vi "Freeze.vi"(8 "Error In":errorcluster, 9 "Waveforms in":waveform(dbl)[](array[waveform]), 10 "Freeze":bool) -> (0 "Error Out":errorcluster, 1 "Waveforms out":waveform(dbl)[](array[waveform]))   [LabVIEW 2017]
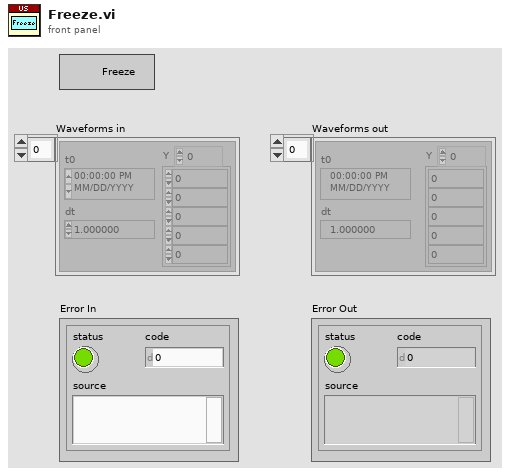
[diagram p1: front panel]
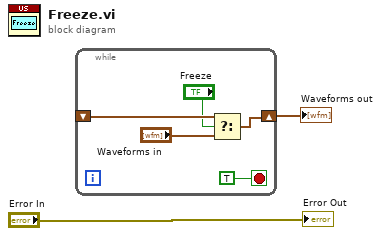
[diagram p0: block diagram]
diagram:
  n1 = while {
    shift-right: [w5] -> w2
    shift-left: _ -> [w6]
    stop <- TRUE stop-if-true
    n2 = Select(t=w6, s="Freeze", f="Waveforms in") -> (s? t:f=w5:waveform(dbl)[])
  }
  "Waveforms out" <- w2
  "Error Out" <- "Error In"
